vi "golpi_mpc_close_octave.vi"(7 "exit command (empty)":string, 8 "error in":errorcluster, 11 "GOLPI ref in":T1={"pipe handle"={"lv_proc.dll file path"=path "", "process instance handle"=[], "debug mode"=FALSE, "debug data"=[]}, "fast read timeout [ms]"=500, "fast read settle time [ms]"=10, "fast read to multiple [ms]"=1, "max elements per input line"=100, "slow read timeout [ms]"=5000, "stdin double format specifier"="%_16e", "max elements per stdout output column"=100, "console mode bitstream"=FALSE, "bitstream first read timeout [ms]"=1000, "bitstream read timeout [ms]"=50, "struct transfer possible"=FALSE}) -> (0 "error out":errorcluster, 2 "exit code":i32, 3 "GOLPI ref out (empty)":T1={"pipe handle"={"lv_proc.dll file path"=path "", "process instance handle"=[], "debug mode"=FALSE, "debug data"=[]}, "fast read timeout [ms]"=500, "fast read settle time [ms]"=10, "fast read to multiple [ms]"=1, "max elements per input line"=100, "slow read timeout [ms]"=5000, "stdin double format specifier"="%_16e", "max elements per stdout output column"=100, "console mode bitstream"=FALSE, "bitstream first read timeout [ms]"=1000, "bitstream read timeout [ms]"=50, "struct transfer possible"=FALSE})   [LabVIEW 2013, in "GOLPI Multi Process.lvlib"]
doc: "Multi-process GOLPI: tries to close Octave. If it's not running it does nothing.\nExit command can be executed before exit.\nThis VI ignores errors and tries to close Octave anyway.\n\nNote: Calling this VI is not necessary because Octave will be terminated when 'golpi_mpc_close_session.vi' is called. It is useful unly when Octave must be terminated and restarted with different GOLPI setup (hide console, change binary path, ...)."
uses:
  GOLPI Multi Process.lvlib
  GOLPI Library.lvlibp/Public/GOLPI reference Type Def.ctl
  GOLPI Library.lvlibp/LV Process source distribution/Pipe Handle.ctl
  GOLPI Library.lvlibp
  GOLPI Library.lvlibp/LV Process source distribution/LV Process library.lvlib
panel:
  out "not running?":bool
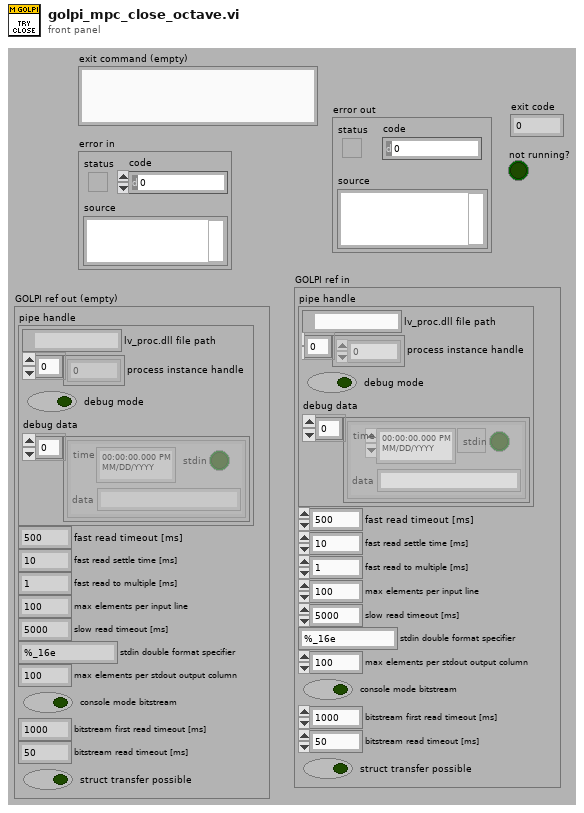
[diagram p1: front panel]
types:
  T1 = typedef "GOLPI Library.lvlibp/GOLPI reference Type Def.ctl" = cluster{"pipe handle":T2, "fast read timeout [ms]":u32, "fast read settle time [ms]":u32, "fast read to multiple [ms]":u32, "max elements per input line":u32, "slow read timeout [ms]":u32, "stdin double format specifier":string, "max elements per stdout output column":u32, "console mode bitstream":bool, "bitstream first read timeout [ms]":u32, "bitstream read timeout [ms]":u32, "struct transfer possible":bool}
  T2 = typedef "GOLPI Library.lvlibp/LV Process library.lvlib/Pipe Handle.ctl" = cluster{"lv_proc.dll file path":path, "process instance handle":u32[], "debug mode":bool, "debug data":cluster{"time":timestamp, "stdin":bool, "data":string}[]}
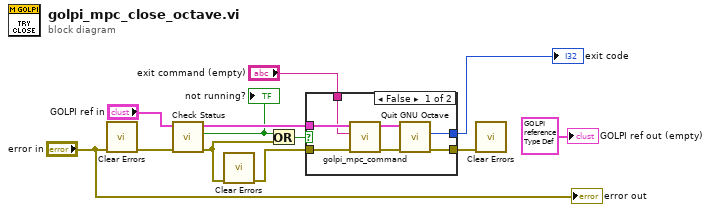
[diagram p0: block diagram]
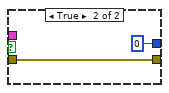
[diagram p2: hidden frame]
diagram:
  n1 = call <vilib>:"Clear Errors.vi"("error in (no error)"="error in") -> ("error out"=w4:errorcluster)  [unwired: 6 in]
  n2 = call "Check Status.vi"("error in"=w4, "GOLPI ref. in"="GOLPI ref in") -> ("error out"=w7:errorcluster, "exited?"=w9:bool, "GOLPI ref. out"=w11:T1)  [unwired: 7 in]
  "not running?" <- w9
  n3 = call <vilib>:"Clear Errors.vi"("error in (no error)"=w7) -> ("error out"=w10:errorcluster)  [unwired: 6 in]
  n4 = Or(x=w9, y=w7) -> (x .or. y?=w8:bool)
  n5 = case shown="False" w8 {
    tunnel: [w19 0 ("exit code")] -> w12
    tunnel: [w18 w20] -> w5
    tunnel: w11 -> [w14 _]
    tunnel: w10 -> [w15 w20]
    tunnel: "exit command (empty)" -> [w13 _]
    frame False {
      n6 = call "golpi_mpc_command.vi"("error in"=w15, "command"=w13, "GOLPI ref in"=w14) -> ("error out"=w17:errorcluster, "GOLPI ref. out"=w16:T1)  [unwired: 6 in, 1 out]
      n7 = call "Quit GNU Octave.vi"("error in"=w17, "GOLPI ref. in"=w16) -> ("error out"=w18:errorcluster, "exit code"=w19:i32)  [unwired: 8 in]
    }
    frame True {
    }
  }
  "exit code" <- w12
  n8 = call <vilib>:"Clear Errors.vi"("error in (no error)"=w5) -> ()  [unwired: 6 in, 1 out]
  "error out" <- "error in"
  "GOLPI ref out (empty)" <- T1 {"pipe handle"={"lv_proc.dll file path"=path "", "process instance handle"=[], "debug mode"=FALSE, "debug data"=[]}, "fast read timeout [ms]"=0, "fast read settle time [ms]"=0, "fast read to multiple [ms]"=0, "max elements per input line"=0, "slow read timeout [ms]"=0, "stdin double format specifier"="", "max elements per stdout output column"=0, "console mode bitstream"=FALSE, "bitstream first read timeout [ms]"=0, "bitstream read timeout [ms]"=0, "struct transfer possible"=FALSE} ("GOLPI ref in")
